vi "HW_set_IO_ports.vi"(1 "Sync capability":u8, 2 "Sync parameters cluster input":T1={"SYNC configuration"=12, "IO 1 configuration"=1, "IO 2 configuration"=1, "IO 3 configuration"=0, "IO 4 configuration"=0, "Activate ext. RS-232"=0}) -> (0 "Sync parameters cluster output":T1={"SYNC configuration"=12, "IO 1 configuration"=1, "IO 2 configuration"=1, "IO 3 configuration"=0, "IO 4 configuration"=0, "Activate ext. RS-232"=0})   [LabVIEW 2018, in "Tracker.lvlib"]
uses:
  Tracker.lvlib
  <vilib>/Utility/miscctls.llb/LVPointTypeDef.ctl
panel:
  in  "Activate ext. RS-232":bool
  in  "Reset IO":bool
  in  "IO 4 zone":bool
  in  "IO 4 start/stop":bool
  in  "IO 3 zone":bool
  in  "IO 3 start/stop":bool
  in  "IO 2 sync":bool
  in  "IO 2 zone":bool=TRUE
  in  "IO 2 start/stop":bool
  in  "IO 1 sync":bool
  in  "IO 1 zone":bool=TRUE
  in  "IO 1 start/stop":bool
  in  "IO 4":u8(slide)=1 scale=0.0..1.0
  in  "IO 3":u8(slide)=1 scale=0.0..1.0
  in  "IO 2":u8(slide) scale=0.0..1.0
  in  "Exit":bool
  in  "Save Settings":bool
  in  "IO 1":u8(slide) scale=0.0..1.0
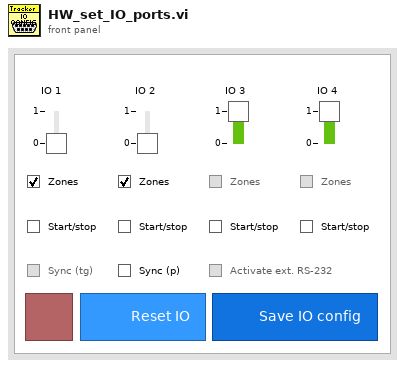
[diagram p1: front panel]
types:
  T1 = cluster{"SYNC configuration":u16, "IO 1 configuration":u16, "IO 2 configuration":u16, "IO 3 configuration":u16, "IO 4 configuration":u16, "Activate ext. RS-232":u16}
  T2 = typedef "LVPointTypeDef.ctl" = cluster{"Horizontal":i16, "Vertical":i16}
  T3 = enum8{"Enabled", "Disabled", "Disabled and Grayed Out"}
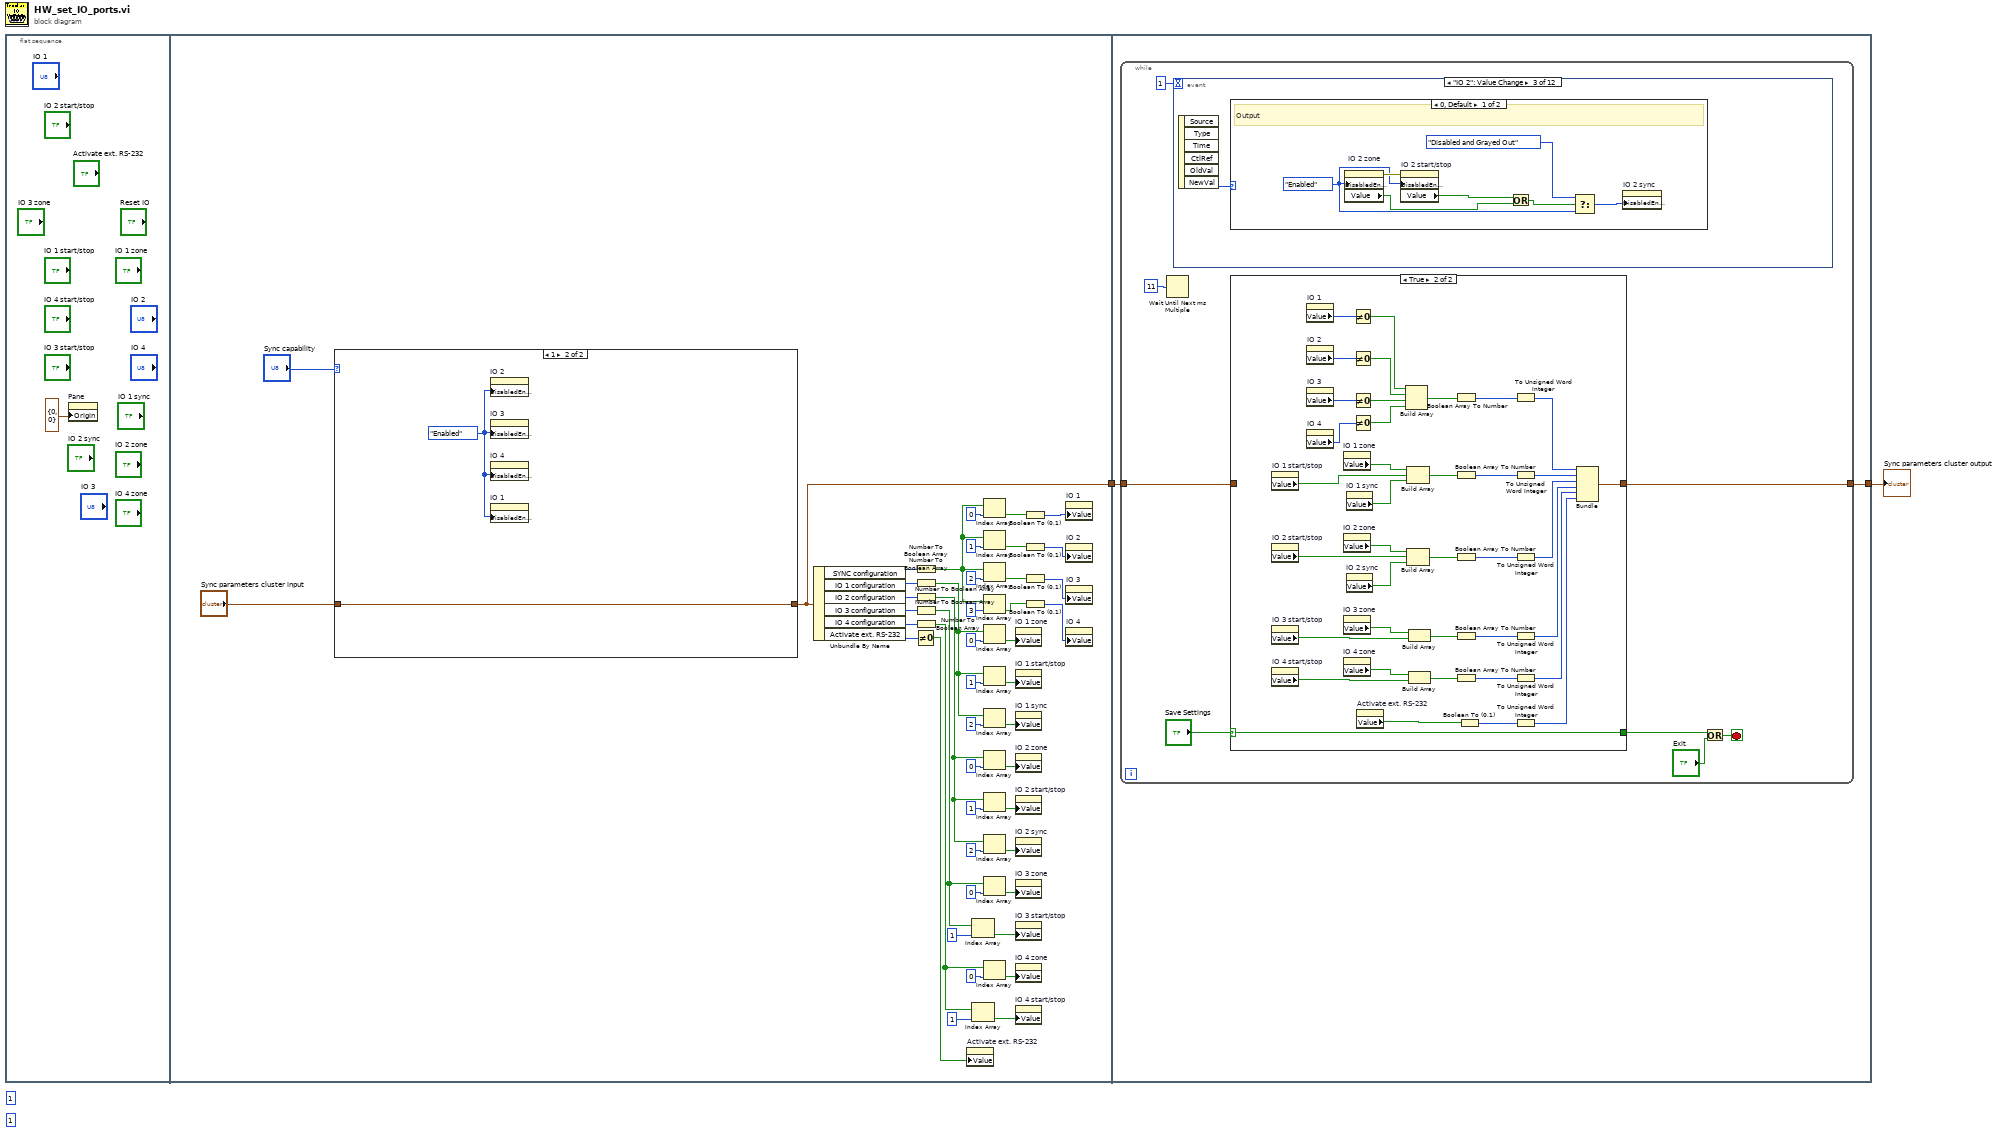
[diagram p0: block diagram]
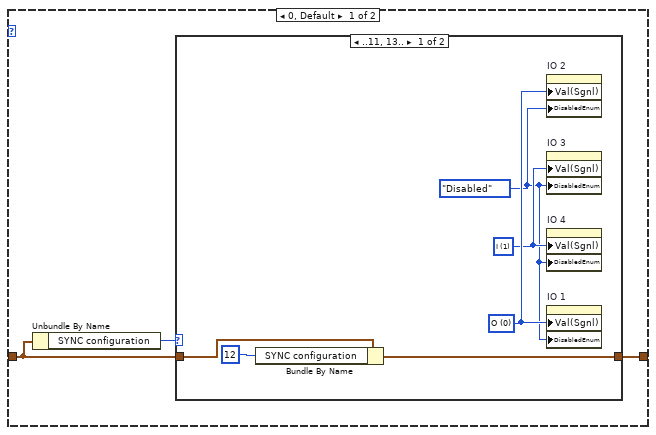
[diagram p2: hidden frame]
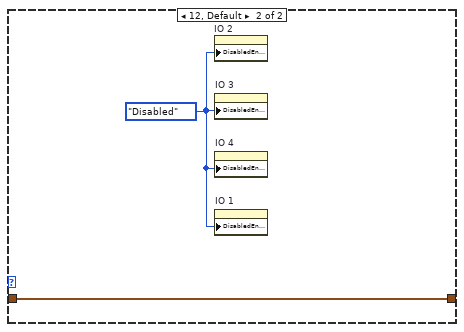
[diagram p3: hidden frame]
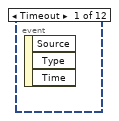
[diagram p5: hidden frame]
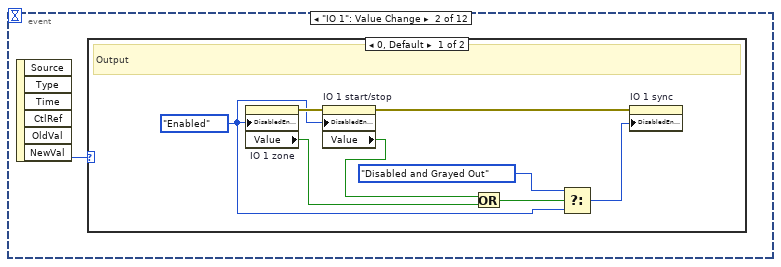
[diagram p6: hidden frame]
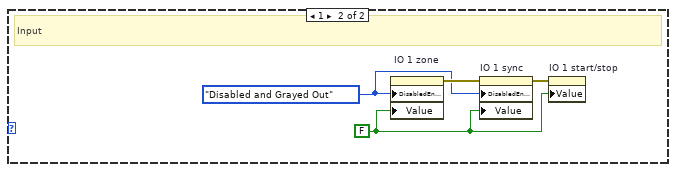
[diagram p7: hidden frame]
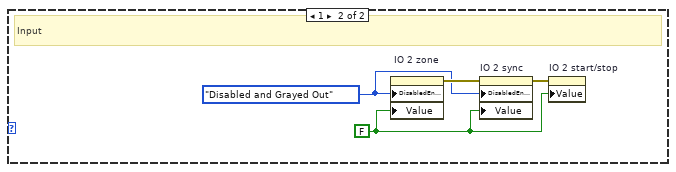
[diagram p8: hidden frame]
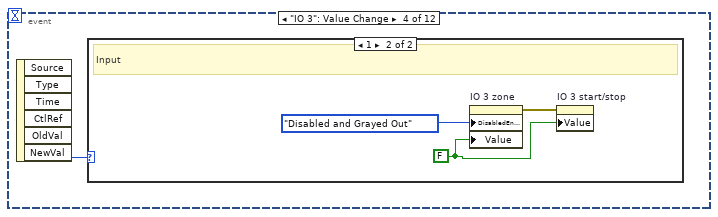
[diagram p9: hidden frame]
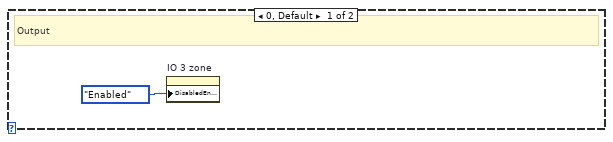
[diagram p10: hidden frame]
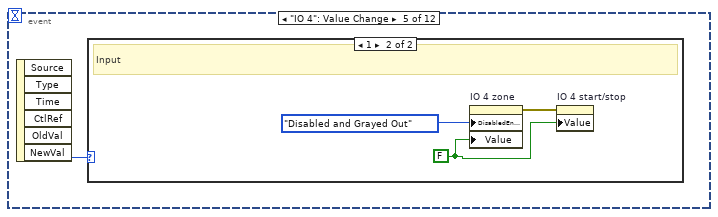
[diagram p11: hidden frame]
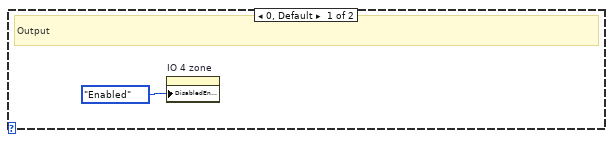
[diagram p12: hidden frame]
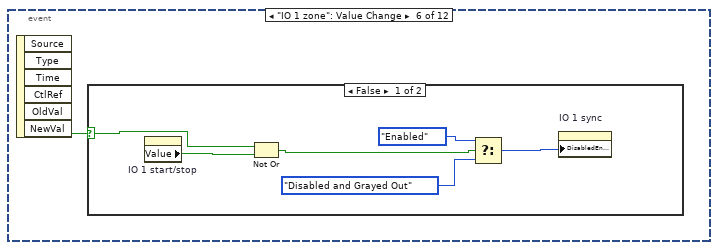
[diagram p13: hidden frame]
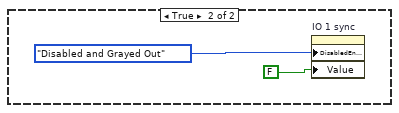
[diagram p14: hidden frame]
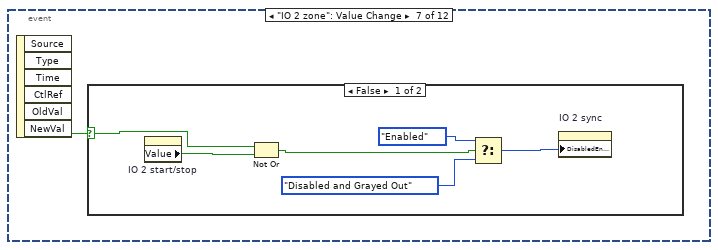
[diagram p15: hidden frame]
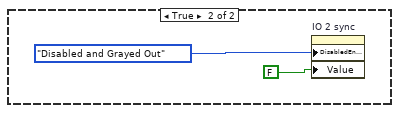
[diagram p16: hidden frame]
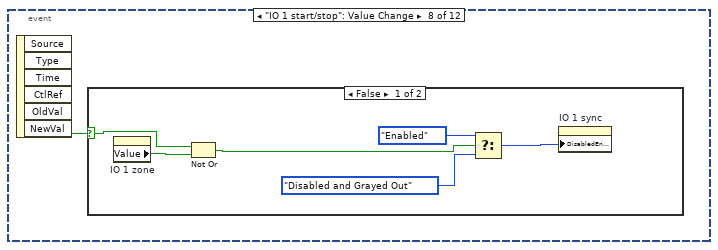
[diagram p17: hidden frame]
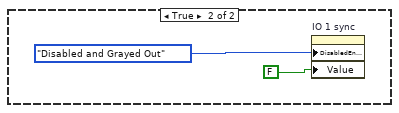
[diagram p18: hidden frame]
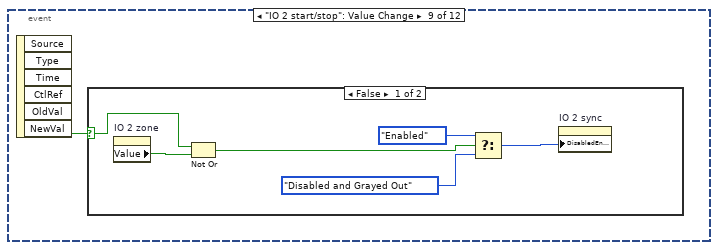
[diagram p19: hidden frame]
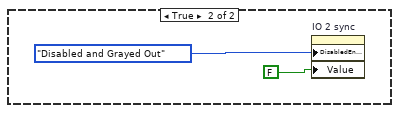
[diagram p20: hidden frame]
diagram:
  (unwired) 1 ("index")
  (unwired) 1 ("index")
  n1 = flat-sequence {
    tunnel: [w6] -> w2
    tunnel: [w65] -> w1
    tunnel: w2 -> [w64]
    frame #0 {
      n2 = property on="Pane" class="Pane"("Origin"=T2 {"Horizontal"=0, "Vertical"=0}) -> ()  [unwired: 2 in, 2 out]
    }
    frame #1 {
      n3 = case shown="1" "Sync capability" {
        tunnel: "Sync parameters cluster input" -> [w52 w63]
        tunnel: [w51 w63] -> w6
        frame 0, Default {
          n4 = Unbundle By Name(w52) -> ("SYNC configuration"=w53:u16)
          n5 = case shown="..11, 13.." w53 {
            tunnel: [w58 w61] -> w51
            tunnel: w52 -> [w59 w61]
            frame ..11, 13.. {
              w54 = T3."Disabled" ("Disabled")
              w55 = u8 1 items=["I"=1, "O"=0] ("IO 3")
              w56 = u8 0 items=["I"=1, "O"=0] ("IO 1")
              n6 = Bundle By Name(cluster=w59, "SYNC configuration"=u16 12) -> (w58:T1)
              n7 = property on="IO 2" class="Slide (strict)"("Val(Sgnl)"=w56, "DisabledEnum"=w54) -> ()  [unwired: 2 in, 2 out]
              n8 = property on="IO 3" class="Slide (strict)"("Val(Sgnl)"=w55, "DisabledEnum"=w54) -> ()  [unwired: 2 in, 2 out]
              n9 = property on="IO 4" class="Slide (strict)"("Val(Sgnl)"=w55, "DisabledEnum"=w54) -> ()  [unwired: 2 in, 2 out]
              n10 = property on="IO 1" class="Slide (strict)"("Val(Sgnl)"=w56, "DisabledEnum"=w54) -> ()  [unwired: 2 in, 2 out]
            }
            frame 12, Default {
              w60 = T3."Disabled" ("Disabled")
              n11 = property on="IO 2" class="Slide (strict)"("DisabledEnum"=w60) -> ()  [unwired: 2 in, 2 out]
              n12 = property on="IO 3" class="Slide (strict)"("DisabledEnum"=w60) -> ()  [unwired: 2 in, 2 out]
              n13 = property on="IO 4" class="Slide (strict)"("DisabledEnum"=w60) -> ()  [unwired: 2 in, 2 out]
              n14 = property on="IO 1" class="Slide (strict)"("DisabledEnum"=w60) -> ()  [unwired: 2 in, 2 out]
            }
          }
        }
        frame 1 {
          w62 = T3."Enabled" ("Disabled")
          n15 = property on="IO 2" class="Slide (strict)"("DisabledEnum"=w62) -> ()  [unwired: 2 in, 2 out]
          n16 = property on="IO 3" class="Slide (strict)"("DisabledEnum"=w62) -> ()  [unwired: 2 in, 2 out]
          n17 = property on="IO 4" class="Slide (strict)"("DisabledEnum"=w62) -> ()  [unwired: 2 in, 2 out]
          n18 = property on="IO 1" class="Slide (strict)"("DisabledEnum"=w62) -> ()  [unwired: 2 in, 2 out]
        }
      }
      n19 = Unbundle By Name(w6) -> ("SYNC configuration"=w50:u16, "IO 1 configuration"=w36:u16, "IO 2 configuration"=w21:u16, "IO 3 configuration"=w12:u16, "IO 4 configuration"=w11:u16, "Activate ext. RS-232"=w10:u16)
      n20 = Not Equal To 0?(x=w10) -> (x != 0?=w9:bool)
      n21 = Number To Boolean Array(number=w50) -> (Boolean array=w49:bool[])
      n22 = Number To Boolean Array(number=w36) -> (Boolean array=w35:bool[])
      n23 = Number To Boolean Array(number=w21) -> (Boolean array=w22:bool[])
      n24 = Number To Boolean Array(number=w12) -> (Boolean array=w20:bool[])
      n25 = Number To Boolean Array(number=w11) -> (Boolean array=w13:bool[])
      n26 = property on="Activate ext. RS-232" class="Bool (strict)"("Value"=w9) -> ()  [unwired: 2 in, 2 out]
      n27 = Index Array(array=w20, index=1) -> (element=w17:bool)
      n28 = Index Array(array=w13, index=1) -> (element=w16:bool)
      n29 = Index Array(array=w49, index=0) -> (element=w44:bool)
      n30 = Index Array(array=w49, index=1) -> (element=w42:bool)
      n31 = Index Array(array=w49, index=2) -> (element=w40:bool)
      n32 = Index Array(array=w49, index=3) -> (element=w38:bool)
      n33 = Index Array(array=w35, index=0) -> (element=w31:bool)
      n34 = Index Array(array=w35, index=1) -> (element=w30:bool)
      n35 = Index Array(array=w35, index=2) -> (element=w29:bool)
      n36 = Index Array(array=w22, index=0) -> (element=w26:bool)
      n37 = Index Array(array=w22, index=1) -> (element=w27:bool)
      n38 = Index Array(array=w22, index=2) -> (element=w28:bool)
      n39 = Index Array(array=w20, index=0) -> (element=w18:bool)
      n40 = Index Array(array=w13, index=0) -> (element=w15:bool)
      n41 = property on="IO 1 zone" class="Bool (strict)"("Value"=w31) -> ()  [unwired: 2 in, 2 out]
      n42 = property on="IO 1 start/stop" class="Bool (strict)"("Value"=w30) -> ()  [unwired: 2 in, 2 out]
      n43 = property on="IO 1 sync" class="Bool (strict)"("Value"=w29) -> ()  [unwired: 2 in, 2 out]
      n44 = property on="IO 2 zone" class="Bool (strict)"("Value"=w26) -> ()  [unwired: 2 in, 2 out]
      n45 = property on="IO 2 start/stop" class="Bool (strict)"("Value"=w27) -> ()  [unwired: 2 in, 2 out]
      n46 = property on="IO 2 sync" class="Bool (strict)"("Value"=w28) -> ()  [unwired: 2 in, 2 out]
      n47 = property on="IO 3 zone" class="Bool (strict)"("Value"=w18) -> ()  [unwired: 2 in, 2 out]
      n48 = property on="IO 3 start/stop" class="Bool (strict)"("Value"=w17) -> ()  [unwired: 2 in, 2 out]
      n49 = property on="IO 4 zone" class="Bool (strict)"("Value"=w15) -> ()  [unwired: 2 in, 2 out]
      n50 = property on="IO 4 start/stop" class="Bool (strict)"("Value"=w16) -> ()  [unwired: 2 in, 2 out]
      n51 = Boolean To (0,1)(Boolean=w44) -> (0, 1=w43:i16)
      n52 = Boolean To (0,1)(Boolean=w42) -> (0, 1=w41:i16)
      n53 = Boolean To (0,1)(Boolean=w40) -> (0, 1=w39:i16)
      n54 = Boolean To (0,1)(Boolean=w38) -> (0, 1=w37:i16)
      n55 = property on="IO 1" class="Slide (strict)"("Value"=w43) -> ()  [unwired: 2 in, 2 out]
      n56 = property on="IO 2" class="Slide (strict)"("Value"=w41) -> ()  [unwired: 2 in, 2 out]
      n57 = property on="IO 3" class="Slide (strict)"("Value"=w39) -> ()  [unwired: 2 in, 2 out]
      n58 = property on="IO 4" class="Slide (strict)"("Value"=w37) -> ()  [unwired: 2 in, 2 out]
    }
    frame #2 {
      n59 = while {
        tunnel: [w67] -> w65
        tunnel: w64 -> [w66]
        stop <- w70 stop-if-true
        n60 = Wait Until Next ms Multiple(millisecond multiple=u32 11) -> ()  [unwired: 1 out]
        n61 = event shown="[2] \"IO 2\": Value Change" {
          selector: _ -> [_ _ _ _ _ _ _ _ _ _ _ _]
          dyn-events: _ -> [_ _ _ _ _ _ _ _ _ _ _ _]
          timeout: 1 -> [_ _ _ _ _ _ _ _ _ _ _ _]
          event Timeout {
            n62 = event-data() -> ()  [unwired: 1 in, 3 out]
          }
          event "IO 1": Value Change {
            n63 = event-data() -> ("NewVal"=w114:u8)  [unwired: 1 in, 5 out]
            n64 = case shown="0, Default" w114 {
              frame 0, Default {
                w118 = T3."Enabled" ("Disabled")
                # "Output"
                n65 = property on="IO 1 zone" class="Bool (strict)"("DisabledEnum"=w118) -> (error out=w122:errorcluster, "Value"=w120:bool)  [unwired: 2 in, 1 out]
                n66 = property on="IO 1 start/stop" class="Bool (strict)"(error in=w122, "DisabledEnum"=w118) -> (error out=w115:errorcluster, "Value"=w121:bool)  [unwired: 1 in, 1 out]
                n67 = Or(x=w121, y=w120) -> (x .or. y?=w119:bool)
                n68 = Select(t=T3."Disabled and Grayed Out", s=w119, f=w118) -> (s? t:f=w117:T3)
                n69 = property on="IO 1 sync" class="Bool (strict)"(error in=w115, "DisabledEnum"=w117) -> ()  [unwired: 1 in, 2 out]
              }
              frame 1 {
                w123 = FALSE ("IO 1 std.")
                w125 = T3."Disabled and Grayed Out" ("Disabled")
                # "Input"
                n70 = property on="IO 1 zone" class="Bool (strict)"("DisabledEnum"=w125, "Value"=w123) -> (error out=w126:errorcluster)  [unwired: 2 in, 1 out]
                n71 = property on="IO 1 sync" class="Bool (strict)"(error in=w126, "DisabledEnum"=w125, "Value"=w123) -> (error out=w124:errorcluster)  [unwired: 1 in, 1 out]
                n72 = property on="IO 1 start/stop" class="Bool (strict)"(error in=w124, "Value"=w123) -> ()  [unwired: 1 in, 2 out]
              }
            }
          }
          event "IO 2": Value Change {
            n73 = event-data() -> ("NewVal"=w127:u8)  [unwired: 1 in, 5 out]
            n74 = case shown="0, Default" w127 {
              frame 0, Default {
                w130 = T3."Enabled" ("Disabled")
                # "Output"
                n75 = property on="IO 2 zone" class="Bool (strict)"("DisabledEnum"=w130) -> (error out=w134:errorcluster, "Value"=w132:bool)  [unwired: 2 in, 1 out]
                n76 = property on="IO 2 start/stop" class="Bool (strict)"(error in=w134, "DisabledEnum"=w130) -> ("Value"=w133:bool)  [unwired: 1 in, 2 out]
                n77 = Or(x=w133, y=w132) -> (x .or. y?=w131:bool)
                n78 = Select(t=T3."Disabled and Grayed Out", s=w131, f=w130) -> (s? t:f=w129:T3)
                n79 = property on="IO 2 sync" class="Bool (strict)"("DisabledEnum"=w129) -> ()  [unwired: 2 in, 2 out]
              }
              frame 1 {
                w135 = FALSE ("IO 1 std.")
                w137 = T3."Disabled and Grayed Out" ("Disabled")
                # "Input"
                n80 = property on="IO 2 zone" class="Bool (strict)"("DisabledEnum"=w137, "Value"=w135) -> (error out=w138:errorcluster)  [unwired: 2 in, 1 out]
                n81 = property on="IO 2 sync" class="Bool (strict)"(error in=w138, "DisabledEnum"=w137, "Value"=w135) -> (error out=w136:errorcluster)  [unwired: 1 in, 1 out]
                n82 = property on="IO 2 start/stop" class="Bool (strict)"(error in=w136, "Value"=w135) -> ()  [unwired: 1 in, 2 out]
              }
            }
          }
          event "IO 3": Value Change {
            n83 = event-data() -> ("NewVal"=w139:u8)  [unwired: 1 in, 5 out]
            n84 = case shown="1" w139 {
              frame 0, Default {
                # "Output"
                n85 = property on="IO 3 zone" class="Bool (strict)"("DisabledEnum"=T3."Enabled" ("Disabled")) -> ()  [unwired: 2 in, 2 out]
              }
              frame 1 {
                w141 = FALSE ("IO 1 std.")
                # "Input"
                n86 = property on="IO 3 zone" class="Bool (strict)"("DisabledEnum"=T3."Disabled and Grayed Out" ("Disabled"), "Value"=w141) -> (error out=w142:errorcluster)  [unwired: 2 in, 1 out]
                n87 = property on="IO 3 start/stop" class="Bool (strict)"(error in=w142, "Value"=w141) -> ()  [unwired: 1 in, 2 out]
              }
            }
          }
          event "IO 4": Value Change {
            n88 = event-data() -> ("NewVal"=w144:u8)  [unwired: 1 in, 5 out]
            n89 = case shown="1" w144 {
              frame 0, Default {
                # "Output"
                n90 = property on="IO 4 zone" class="Bool (strict)"("DisabledEnum"=T3."Enabled" ("Disabled")) -> ()  [unwired: 2 in, 2 out]
              }
              frame 1 {
                w146 = FALSE ("IO 1 std.")
                # "Input"
                n91 = property on="IO 4 zone" class="Bool (strict)"("DisabledEnum"=T3."Disabled and Grayed Out" ("Disabled"), "Value"=w146) -> (error out=w147:errorcluster)  [unwired: 2 in, 1 out]
                n92 = property on="IO 4 start/stop" class="Bool (strict)"(error in=w147, "Value"=w146) -> ()  [unwired: 1 in, 2 out]
              }
            }
          }
          event "IO 1 zone": Value Change {
            n93 = event-data() -> ("NewVal"=w149:bool)  [unwired: 1 in, 5 out]
            n94 = case shown="False" w149 {
              selector: w149 -> [w154 _]
              frame False {
                n95 = property on="IO 1 start/stop" class="Bool (strict)"() -> ("Value"=w155:bool)  [unwired: 2 in, 2 out]
                n96 = Not Or(1:w155, 2:w154) -> (0:w153:bool)
                n97 = Select(t=T3."Enabled" ("Disabled"), s=w153, f=T3."Disabled and Grayed Out") -> (s? t:f=w151:T3)
                n98 = property on="IO 1 sync" class="Bool (strict)"("DisabledEnum"=w151) -> ()  [unwired: 2 in, 2 out]
              }
              frame True {
                n99 = property on="IO 1 sync" class="Bool (strict)"("DisabledEnum"=T3."Disabled and Grayed Out" ("Disabled"), "Value"=FALSE ("IO 1 sync")) -> ()  [unwired: 2 in, 2 out]
              }
            }
          }
          event "IO 2 zone": Value Change {
            n100 = event-data() -> ("NewVal"=w158:bool)  [unwired: 1 in, 5 out]
            n101 = case shown="False" w158 {
              selector: w158 -> [w163 _]
              frame False {
                n102 = property on="IO 2 start/stop" class="Bool (strict)"() -> ("Value"=w164:bool)  [unwired: 2 in, 2 out]
                n103 = Not Or(1:w164, 2:w163) -> (0:w162:bool)
                n104 = Select(t=T3."Enabled" ("Disabled"), s=w162, f=T3."Disabled and Grayed Out") -> (s? t:f=w160:T3)
                n105 = property on="IO 2 sync" class="Bool (strict)"("DisabledEnum"=w160) -> ()  [unwired: 2 in, 2 out]
              }
              frame True {
                n106 = property on="IO 2 sync" class="Bool (strict)"("DisabledEnum"=T3."Disabled and Grayed Out" ("Disabled"), "Value"=FALSE ("IO 1 sync")) -> ()  [unwired: 2 in, 2 out]
              }
            }
          }
          event "IO 1 start/stop": Value Change {
            n107 = event-data() -> ("NewVal"=w167:bool)  [unwired: 1 in, 5 out]
            n108 = case shown="False" w167 {
              selector: w167 -> [w173 _]
              frame False {
                n109 = property on="IO 1 zone" class="Bool (strict)"() -> ("Value"=w172:bool)  [unwired: 2 in, 2 out]
                n110 = Not Or(1:w172, 2:w173) -> (0:w171:bool)
                n111 = Select(t=T3."Enabled" ("Disabled"), s=w171, f=T3."Disabled and Grayed Out") -> (s? t:f=w168:T3)
                n112 = property on="IO 1 sync" class="Bool (strict)"("DisabledEnum"=w168) -> ()  [unwired: 2 in, 2 out]
              }
              frame True {
                n113 = property on="IO 1 sync" class="Bool (strict)"("DisabledEnum"=T3."Disabled and Grayed Out" ("Disabled"), "Value"=FALSE ("IO 1 sync")) -> ()  [unwired: 2 in, 2 out]
              }
            }
          }
          event "IO 2 start/stop": Value Change {
            n114 = event-data() -> ("NewVal"=w176:bool)  [unwired: 1 in, 5 out]
            n115 = case shown="False" w176 {
              selector: w176 -> [w182 _]
              frame False {
                n116 = property on="IO 2 zone" class="Bool (strict)"() -> ("Value"=w181:bool)  [unwired: 2 in, 2 out]
                n117 = Not Or(1:w181, 2:w182) -> (0:w180:bool)
                n118 = Select(t=T3."Enabled" ("Disabled"), s=w180, f=T3."Disabled and Grayed Out") -> (s? t:f=w177:T3)
                n119 = property on="IO 2 sync" class="Bool (strict)"("DisabledEnum"=w177) -> ()  [unwired: 2 in, 2 out]
              }
              frame True {
                n120 = property on="IO 2 sync" class="Bool (strict)"("DisabledEnum"=T3."Disabled and Grayed Out" ("Disabled"), "Value"=FALSE ("IO 1 sync")) -> ()  [unwired: 2 in, 2 out]
              }
            }
          }
          event "IO 1 sync": Value Change {
            n121 = event-data() -> ("NewVal"=w185:bool)  [unwired: 1 in, 5 out]
            n122 = case shown="True" w185 {
              frame False {
                w187 = T3."Enabled" ("Disabled")
                n123 = property on="IO 1 zone" class="Bool (strict)"("DisabledEnum"=w187) -> (error out=w186:errorcluster)  [unwired: 2 in, 1 out]
                n124 = property on="IO 1 start/stop" class="Bool (strict)"(error in=w186, "DisabledEnum"=w187) -> ()  [unwired: 1 in, 2 out]
              }
              frame True {
                w188 = T3."Disabled and Grayed Out" ("Disabled")
                w189 = FALSE ("IO 1 zone")
                n125 = property on="IO 1 start/stop" class="Bool (strict)"("DisabledEnum"=w188, "Value"=w189) -> ()  [unwired: 2 in, 2 out]
                n126 = property on="IO 1 zone" class="Bool (strict)"("DisabledEnum"=w188, "Value"=w189) -> ()  [unwired: 2 in, 2 out]
              }
            }
          }
          event "IO 2 sync": Value Change {
            n127 = event-data() -> ("NewVal"=w190:bool)  [unwired: 1 in, 5 out]
            n128 = case shown="False" w190 {
              frame False {
                w192 = T3."Enabled" ("Disabled")
                n129 = property on="IO 2 zone" class="Bool (strict)"("DisabledEnum"=w192) -> (error out=w191:errorcluster)  [unwired: 2 in, 1 out]
                n130 = property on="IO 2 start/stop" class="Bool (strict)"(error in=w191, "DisabledEnum"=w192) -> ()  [unwired: 1 in, 2 out]
              }
              frame True {
                w193 = T3."Disabled and Grayed Out" ("Disabled")
                w194 = FALSE ("IO 1 zone")
                n131 = property on="IO 2 start/stop" class="Bool (strict)"("DisabledEnum"=w193, "Value"=w194) -> ()  [unwired: 2 in, 2 out]
                n132 = property on="IO 2 zone" class="Bool (strict)"("DisabledEnum"=w193, "Value"=w194) -> ()  [unwired: 2 in, 2 out]
              }
            }
          }
          event "Reset IO": Value Change {
            w215 = u8 1 ("Value (Signaling)")
            w216 = u8 0 ("Value (Signaling)")
            n133 = event-data() -> ()  [unwired: 1 in, 6 out]
            n134 = property on="IO 1" class="Slide (strict)"("Val(Sgnl)"=w216) -> (error out=w214:errorcluster)  [unwired: 2 in, 1 out]
            n135 = property on="IO 2" class="Slide (strict)"("Val(Sgnl)"=w216) -> (error out=w207:errorcluster)  [unwired: 2 in, 1 out]
            n136 = property on="IO 1 zone" class="Bool (strict)"(error in=w214, "Val(Sgnl)"=TRUE ("Value (Signaling)")) -> (error out=w213:errorcluster)  [unwired: 1 in, 1 out]
            n137 = property on="IO 2 zone" class="Bool (strict)"(error in=w207, "Val(Sgnl)"=TRUE ("Value (Signaling)")) -> (error out=w208:errorcluster)  [unwired: 1 in, 1 out]
            n138 = property on="IO 3" class="Slide (strict)"("Val(Sgnl)"=w215) -> (error out=w205:errorcluster)  [unwired: 2 in, 1 out]
            n139 = property on="IO 4" class="Slide (strict)"("Val(Sgnl)"=w215) -> (error out=w203:errorcluster)  [unwired: 2 in, 1 out]
            n140 = property on="IO 1 start/stop" class="Bool (strict)"(error in=w213, "Val(Sgnl)"=FALSE ("Value (Signaling)")) -> (error out=w202:errorcluster)  [unwired: 1 in, 1 out]
            n141 = property on="IO 2 start/stop" class="Bool (strict)"(error in=w208, "Val(Sgnl)"=FALSE ("Value (Signaling)")) -> (error out=w201:errorcluster)  [unwired: 1 in, 1 out]
            n142 = property on="IO 3 start/stop" class="Bool (strict)"(error in=w205, "Val(Sgnl)"=FALSE ("Value (Signaling)")) -> (error out=w200:errorcluster)  [unwired: 1 in, 1 out]
            n143 = property on="IO 4 start/stop" class="Bool (strict)"(error in=w203, "Val(Sgnl)"=FALSE ("Value (Signaling)")) -> (error out=w199:errorcluster)  [unwired: 1 in, 1 out]
            n144 = Merge Errors(w202, w201, w200, w199) -> (w198:errorcluster)
            n145 = property on="Reset IO" class="Bool (strict)"(error in=w198, "Value"=FALSE ("Reset IO")) -> (error out=w195:errorcluster)  [unwired: 1 in, 1 out]
            n146 = property on="Activate ext. RS-232" class="Bool (strict)"(error in=w195, "Value"=FALSE ("Activate ext. RS-232")) -> ()  [unwired: 1 in, 2 out]
          }
        }
        n147 = case shown="True" "Save Settings" {
          selector: "Save Settings" -> [w75 w103]
          tunnel: [w75 w103] -> w68
          tunnel: [w74 w86] -> w67
          tunnel: w66 -> [w74 _]
          frame False {
          }
          frame True {
            n148 = property on="IO 1 start/stop" class="Bool (strict)"() -> ("Value"=w101:bool)  [unwired: 2 in, 2 out]
            n149 = property on="IO 2 start/stop" class="Bool (strict)"() -> ("Value"=w96:bool)  [unwired: 2 in, 2 out]
            n150 = property on="IO 3 start/stop" class="Bool (strict)"() -> ("Value"=w93:bool)  [unwired: 2 in, 2 out]
            n151 = property on="IO 4 start/stop" class="Bool (strict)"() -> ("Value"=w90:bool)  [unwired: 2 in, 2 out]
            n152 = property on="IO 1" class="Slide (strict)"() -> ("Value"=w113:u8)  [unwired: 2 in, 2 out]
            n153 = property on="IO 2" class="Slide (strict)"() -> ("Value"=w112:u8)  [unwired: 2 in, 2 out]
            n154 = property on="IO 3" class="Slide (strict)"() -> ("Value"=w111:u8)  [unwired: 2 in, 2 out]
            n155 = property on="IO 4" class="Slide (strict)"() -> ("Value"=w110:u8)  [unwired: 2 in, 2 out]
            n156 = property on="IO 1 zone" class="Bool (strict)"() -> ("Value"=w102:bool)  [unwired: 2 in, 2 out]
            n157 = property on="IO 2 zone" class="Bool (strict)"() -> ("Value"=w95:bool)  [unwired: 2 in, 2 out]
            n158 = property on="IO 3 zone" class="Bool (strict)"() -> ("Value"=w92:bool)  [unwired: 2 in, 2 out]
            n159 = property on="IO 4 zone" class="Bool (strict)"() -> ("Value"=w91:bool)  [unwired: 2 in, 2 out]
            n160 = property on="IO 1 sync" class="Bool (strict)"() -> ("Value"=w100:bool)  [unwired: 2 in, 2 out]
            n161 = property on="IO 2 sync" class="Bool (strict)"() -> ("Value"=w97:bool)  [unwired: 2 in, 2 out]
            n162 = Not Equal To 0?(x=w113) -> (x != 0?=w109:bool)
            n163 = Not Equal To 0?(x=w112) -> (x != 0?=w108:bool)
            n164 = Not Equal To 0?(x=w111) -> (x != 0?=w107:bool)
            n165 = Not Equal To 0?(x=w110) -> (x != 0?=w106:bool)
            n166 = property on="Activate ext. RS-232" class="Bool (strict)"() -> ("Value"=w87:bool)  [unwired: 2 in, 2 out]
            n167 = Build Array(w109, w108, w107, w106) -> (w105:bool[])
            n168 = Build Array(w102, w101, w100) -> (w99:bool[])
            n169 = Build Array(w95, w96, w97) -> (w98:bool[])
            n170 = Build Array(w92, w93) -> (w94:bool[])
            n171 = Build Array(w91, w90) -> (w89:bool[])
            n172 = Boolean Array To Number(Boolean array=w105) -> (number=w104:u32)
            n173 = Boolean Array To Number(Boolean array=w99) -> (number=w81:u32)
            n174 = Boolean Array To Number(Boolean array=w98) -> (number=w79:u32)
            n175 = Boolean Array To Number(Boolean array=w94) -> (number=w77:u32)
            n176 = Boolean Array To Number(Boolean array=w89) -> (number=w88:u32)
            n177 = Boolean To (0,1)(Boolean=w87) -> (0, 1=w85:i16)
            n178 = To Unsigned Word Integer(number=w104) -> (unsigned 16bit integer=w83:u16)
            n179 = To Unsigned Word Integer(number=w81) -> (unsigned 16bit integer=w80:u16)
            n180 = To Unsigned Word Integer(number=w79) -> (unsigned 16bit integer=w78:u16)
            n181 = To Unsigned Word Integer(number=w77) -> (unsigned 16bit integer=w76:u16)
            n182 = To Unsigned Word Integer(number=w88) -> (unsigned 16bit integer=w82:u16)
            n183 = To Unsigned Word Integer(number=w85) -> (unsigned 16bit integer=w84:u16)
            n184 = Bundle(w83, w80, w78, w76, w82, w84) -> (w86:cluster{u16, u16, u16, u16, u16, u16})  [unwired: 1 in]
          }
        }
        n185 = Or(x=w68, y="Exit") -> (x .or. y?=w70:bool)
      }
    }
  }
  "Sync parameters cluster output" <- w1
